vi "Configure Channel.vi"(8 "error in (no error)":errorcluster, 9 "Channel Config":T1=enum."Disabled", 10 "Channel in":T2, 11 "EPU452 in":refnum<class "EPU452.lvclass">) -> (0 "error out":errorcluster, 2 "Response":string, 3 "EPU452 out":refnum<class "EPU452.lvclass">)   [LabVIEW 2018, in "EPU452.lvclass"]
uses:
  EPU452.lvclass
  Controls/Channels.ctl
  Controls/Channel Config.ctl
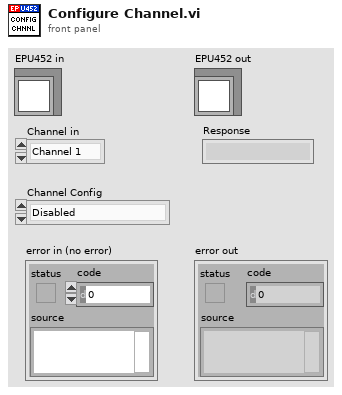
[diagram p1: front panel]
types:
  T1 = typedef "EPU452.lvclass/Channel Config.ctl" = enum16{"Unknown", "Disabled", "Voltmeter", "pH/ISE", "Pt 1k RTD", "10 k Thermistor", "dO2", "Biosensor", "Conductivity"}
  T2 = typedef "EPU452.lvclass/Channels.ctl" = enum16{"Channel 1", "Channel 2", "Channel 3", "Channel 4"}
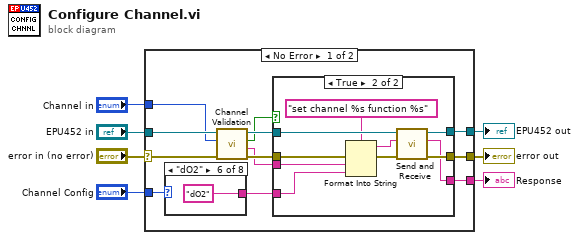
[diagram p0: block diagram]
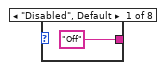
[diagram p2: hidden frame]
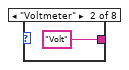
[diagram p3: hidden frame]
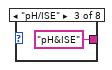
[diagram p4: hidden frame]
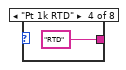
[diagram p5: hidden frame]
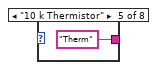
[diagram p6: hidden frame]
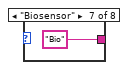
[diagram p7: hidden frame]
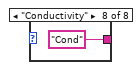
[diagram p8: hidden frame]
diagram:
  n1 = case shown="No Error" "error in (no error)" {
    selector: "error in (no error)" -> [w10 w41]
    tunnel: [w16 w41] -> w6
    tunnel: [w17 w40] -> w4
    tunnel: "EPU452 in" -> [w11 w40]
    tunnel: "Channel in" -> [w9 _]
    tunnel: "Channel Config" -> [w13 _]
    tunnel: [w8 _] -> w1
    frame No Error {
      n2 = case shown="\"dO2\"" w13 {
        tunnel: ["Off" "Volt" "pH&ISE" "RTD" "Therm" "dO2" "Bio" "Cond"] -> w12
        frame "Disabled", Default {
        }
        frame "Voltmeter" {
        }
        frame "pH/ISE" {
        }
        frame "Pt 1k RTD" {
        }
        frame "10 k Thermistor" {
        }
        frame "dO2" {
        }
        frame "Biosensor" {
        }
        frame "Conductivity" {
        }
      }
      n3 = call "Channel Validation.vi"("error in (no error)"=w10, "Channel in"=w9, "EPU452 in"=w11) -> ("error out"=w19:errorcluster, "Channel"=w14:string, "Is Channel Valid?"=w15:bool, "EPU452 out"=w18:refnum<class "EPU452.lvclass">)  [unwired: 5 in]
      n4 = case shown="True" w15 {
        tunnel: w19 -> [w28 w38]
        tunnel: w18 -> [w29 w37]
        tunnel: w14 -> [_ w33]
        tunnel: [w29 w35] -> w17
        tunnel: [w28 w34] -> w16
        tunnel: w12 -> [_ w32]
        tunnel: [_ w30] -> w8
        frame False {
        }
        frame True {
          n5 = Format Into String(format string="set channel %s function %s", error in=w38, w33, w32) -> (resulting string=w31:string, error out=w39:errorcluster)  [unwired: 1 in]
          n6 = call "Send and Receive.vi"("error in (no error)"=w39, "Command"=w31, "EPU452 in"=w37) -> ("error out"=w34:errorcluster, "Response"=w30:string, "EPU452 out"=w35:refnum<class "EPU452.lvclass">)  [unwired: 6 in]
        }
      }
    }
    frame Error {
    }
  }
  "error out" <- w6
  "EPU452 out" <- w4
  "Response" <- w1
